vi "Calibration Get Channels DAQ Parameters.vi"(8 "error in (no error)":errorcluster, 11 "Main":string) -> (0 "error out":errorcluster, 2 "Single Channel DAQ Parameters":T1, 3 "DAQ Parameters":T1[](array[typedef]))   [LabVIEW 2017, in "SQLite.lvclass"]
doc: "in put the sensors name list \nget each channel MuliplyFactor ,RawPrecision, PhysicalPrecision"
uses:
  SQLite.lvclass
  DAQParameters.ctl
  Order By.ctl
  <userlib>/sushu/sushu.lvlib
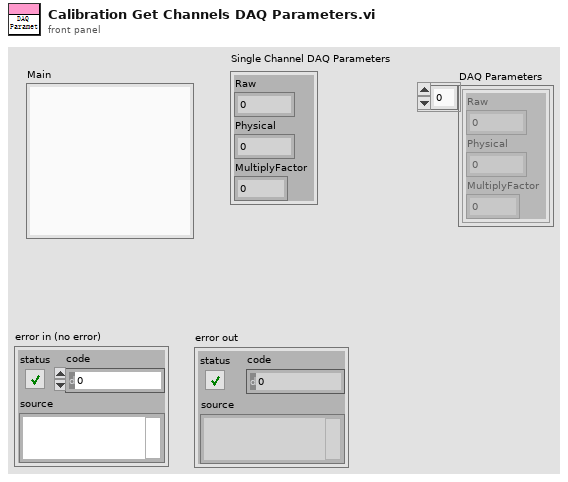
[diagram p1: front panel]
types:
  T1 = typedef "SQLite.lvclass/DAQParameters.ctl" = cluster{"Raw":i16, "Physical":i16, "MultiplyFactor":dbl}
  T2 = typedef "SQLite.lvclass/Order By.ctl" = cluster{"Attach":bool, "Column index":i32}
  T3 = cluster{"[0]":T1, "[1]":T1, "[2]":T1, "[3]":T1, "[4]":T1, "[5]":T1, "[6]":T1, "[7]":T1, "[8]":T1, "[9]":T1, "[10]":T1, "[11]":T1, "[12]":T1, "[13]":T1, "[14]":T1}
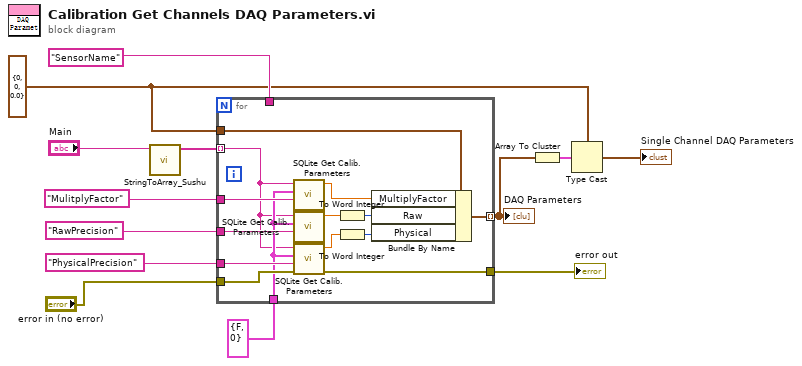
[diagram p0: block diagram]
diagram:
  w3 = T1 {"Raw"=0, "Physical"=0, "MultiplyFactor"=0.0} ("DAQParameters")
  n1 = call <userlib>:"StringToArray_Sushu.vi"("State Queue"="Main") -> ("Array"=w12:string[])  [unwired: 8 in, 2 out]
  n2 = for {
    tunnel: "SensorName" ("Main") -> [_]
    tunnel: "PhysicalPrecision" ("VariableName") -> [w22]
    tunnel: "RawPrecision" ("VariableName") -> [w21]
    tunnel: "MulitplyFactor" ("VariableName") -> [w20]
    tunnel: [w19] -> w4 mode=indexing
    tunnel: w3 -> [w18]
    tunnel: "error in (no error)" -> [w17]
    tunnel: [w16] -> w6
    tunnel: T2 {"Attach"=FALSE, "Column index"=0} ("Order By") -> [w15]
    tunnel: w12 -> [w14] mode=indexing
    n3 = call "SQLite Get Calib.Parameters.vi"("VariableName"=w20, "Order By"=w15, "Main"=w14) -> ("DBL Value"=w23:dbl)  [unwired: 3 in, 5 out]
    n4 = call "SQLite Get Calib.Parameters.vi"("VariableName"=w21, "Order By"=w15, "Main"=w14) -> ("DBL Value"=w27:dbl)  [unwired: 3 in, 5 out]
    n5 = call "SQLite Get Calib.Parameters.vi"("error in (no error)"=w17, "VariableName"=w22, "Order By"=w15, "Main"=w14) -> ("error out"=w16:errorcluster, "DBL Value"=w26:dbl)  [unwired: 2 in, 4 out]
    n6 = To Word Integer(number=w27) -> (16bit integer=w25:i16)
    n7 = To Word Integer(number=w26) -> (16bit integer=w24:i16)
    n8 = Bundle By Name(cluster=w18, "MultiplyFactor"=w23, "Raw"=w25, "Physical"=w24) -> (w19:T1)
  }
  "error out" <- w6
  "DAQ Parameters" <- w4
  n9 = Array To Cluster(array=w4) -> (cluster=w5:T3)
  n10 = Type Cast(type=w3, x=w5) -> (*(type *) &x=→"Single Channel DAQ Parameters":T1)
